vi "rethinkdb_tcp_parse_errors.vi"(8 "error in (no error)":errorcluster, 11 "messages":string[](array[string])) -> (0 "error out":errorcluster, 3 "remaining messages":string[](array[string]))   [LabVIEW 2017]
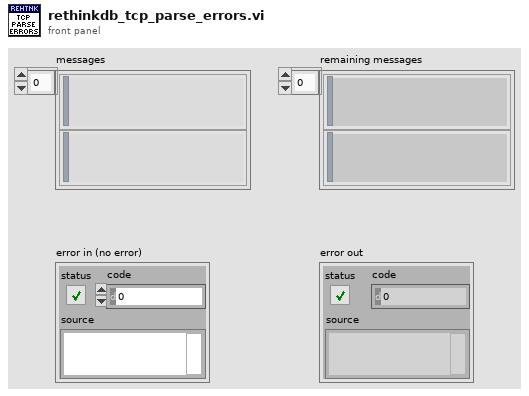
[diagram p1: front panel]
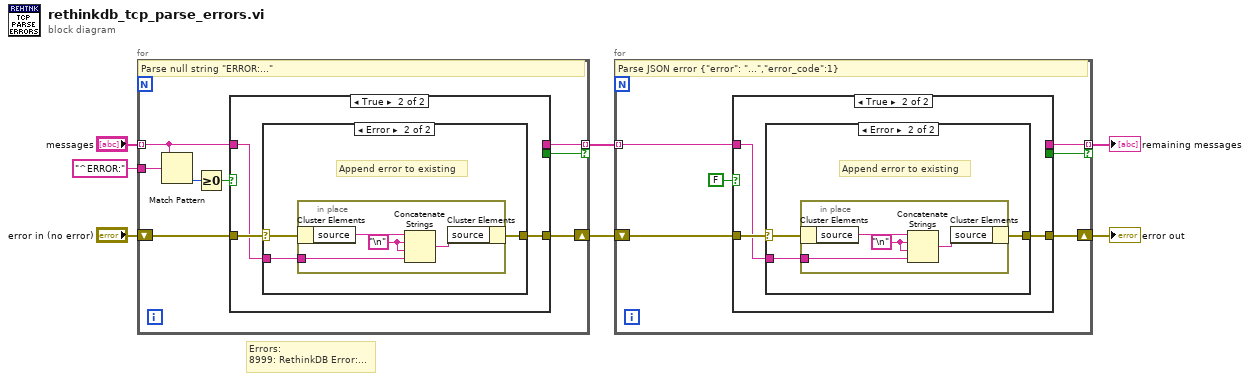
[diagram p0: block diagram]
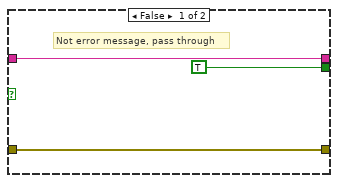
[diagram p2: hidden frame]
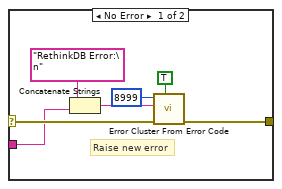
[diagram p3: hidden frame]
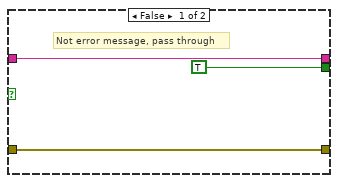
[diagram p4: hidden frame]
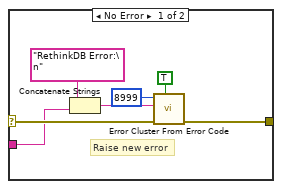
[diagram p5: hidden frame]
diagram:
  # "Errors:\n8999: RethinkDB Error:..."
  n1 = for {
    tunnel: "^ERROR:" -> [w15]
    tunnel: "messages" -> [w9] mode=indexing
    tunnel: [w8] -> w3 mode=indexing if=w11
    shift-right: [w10] -> w4
    shift-left: "error in (no error)" -> [w12]
    # "Parse null string \"ERROR:...\""
    n2 = Match Pattern(string=w9, regular expression=w15) -> (offset past match=w14:i32)  [unwired: 1 in, 3 out]
    n3 = Greater Or Equal To 0?(x=w14) -> (x >= 0?=w13:bool)
    n4 = case shown="True" w13 {
      tunnel: w12 -> [w16 w21]
      tunnel: [TRUE _] -> w11
      tunnel: w9 -> [w17 w19]
      tunnel: [w16 w20] -> w10
      tunnel: [w17 _] -> w8
      frame False {
        # "Not error message, pass through"
      }
      frame True {
        n5 = case shown="Error" w21 {
          selector: w21 -> [w28 w31]
          tunnel: [w25 w30] -> w20
          tunnel: w19 -> [w23 w29]
          frame No Error {
            # "Raise new error"
            n6 = Concatenate Strings("RethinkDB Error:\n" ("error message (\"\")"), w23) -> (w22:string)
            n7 = call <vilib>:"Error Cluster From Error Code.vi"("show call chain? (False)"=TRUE, "error in (no error)"=w28, "error message (\"\")"=w22, "error code (0)"=8999) -> ("error out"=w25:errorcluster)  [unwired: 5 in]
          }
          frame Error {
            # "Append error to existing"
            n8 = in-place {
              in-place-border: w29 -> [w33]
              w32 = "\n"
              n9 = in-place-cluster #1(w31) -> ("source"=w35:string)
              n10 = Concatenate Strings(w35, w32, w32, w33) -> (w34:string)
              n11 = in-place-cluster #1("source"=w34) -> (w30:errorcluster)
            }
          }
        }
      }
    }
  }
  n12 = for {
    tunnel: w3 -> [w38] mode=indexing
    tunnel: [w37] -> w1 mode=indexing if=w40
    shift-right: [w39] -> w2
    shift-left: w4 -> [w41]
    # "Parse JSON error {\"error\": \"...\",\"error_code\":1}"
    n13 = case shown="True" FALSE {
      tunnel: w41 -> [w42 w47]
      tunnel: [TRUE _] -> w40
      tunnel: w38 -> [w43 w45]
      tunnel: [w42 w46] -> w39
      tunnel: [w43 _] -> w37
      frame False {
        # "Not error message, pass through"
      }
      frame True {
        n14 = case shown="Error" w47 {
          selector: w47 -> [w54 w57]
          tunnel: [w51 w56] -> w46
          tunnel: w45 -> [w49 w55]
          frame No Error {
            # "Raise new error"
            n15 = Concatenate Strings("RethinkDB Error:\n" ("error message (\"\")"), w49) -> (w48:string)
            n16 = call <vilib>:"Error Cluster From Error Code.vi"("show call chain? (False)"=TRUE, "error in (no error)"=w54, "error message (\"\")"=w48, "error code (0)"=8999) -> ("error out"=w51:errorcluster)  [unwired: 5 in]
          }
          frame Error {
            # "Append error to existing"
            n17 = in-place {
              in-place-border: w55 -> [w59]
              w58 = "\n"
              n18 = in-place-cluster #2(w57) -> ("source"=w61:string)
              n19 = Concatenate Strings(w61, w58, w58, w59) -> (w60:string)
              n20 = in-place-cluster #2("source"=w60) -> (w56:errorcluster)
            }
          }
        }
      }
    }
  }
  "error out" <- w2
  "remaining messages" <- w1
